vi "Supplementary Fig.15-2.vi"() -> ()   [LabVIEW 2018]
panel:
  out "files":string[](array[string])=["3rd-no3_th0_20191112171700-ext.FIRE", "3rd-no3_th0_20191112171706-ext.FIRE", "3rd-no3_th0_20191112171712-ext.FIRE", "3rd-no3_th0_20191112171717-ext.FIRE", "3rd-no3_th0_20191112171723-ext.FIRE", "3rd-no3_th0_20191112171728-ext.FIRE", "3rd-no3_th0_20191112171733-ext.FIRE", "3rd-no3_th0_20191112171739-ext.FIRE", "3rd-no3_th0_20191112171744-ext.FIRE", "3rd-no3_th0_20191112171750-ext.FIRE", "3rd-no3_th0_20191112171756-ext.FIRE", "3rd-no3_th0_20191112171801-ext.FIRE", "3rd-no3_th0_20191112171807-ext.FIRE", "3rd-no3_th0_20191112171813-ext.FIRE", "3rd-no3_th0_20191112171819-ext.FIRE", "3rd-no3_th0_20191112171824-ext.FIRE", "3rd-no3_th0_20191112171829-ext.FIRE", "3rd-no3_th0_20191112171835-ext.FIRE", "3rd-no3_th0_20191112171840-ext.FIRE", "3rd-no3_th0_20191112171846-ext.FIRE", "3rd-no3_th0_20191112171851-ext.FIRE", "3rd-no3_th0_20191112171857-ext.FIRE"]
  out "widths [um] (red x, red y, green x, green y)":dbl[][](array[numeric])
  in  "Array 3":T1(array[cluster])=[{"index"=6, "upper limit"=3.0, "lower limit"=1e-06, "Boolean"=TRUE}, {"index"=10, "upper limit"=3.0, "lower limit"=1e-06, "Boolean"=TRUE}, {"index"=14, "upper limit"=3.0, "lower limit"=1e-06, "Boolean"=TRUE}, {"index"=18, "upper limit"=3.0, "lower limit"=1e-06, "Boolean"=TRUE}]
  in  "file type":string=".info"
  in  "filepath (.info)":path
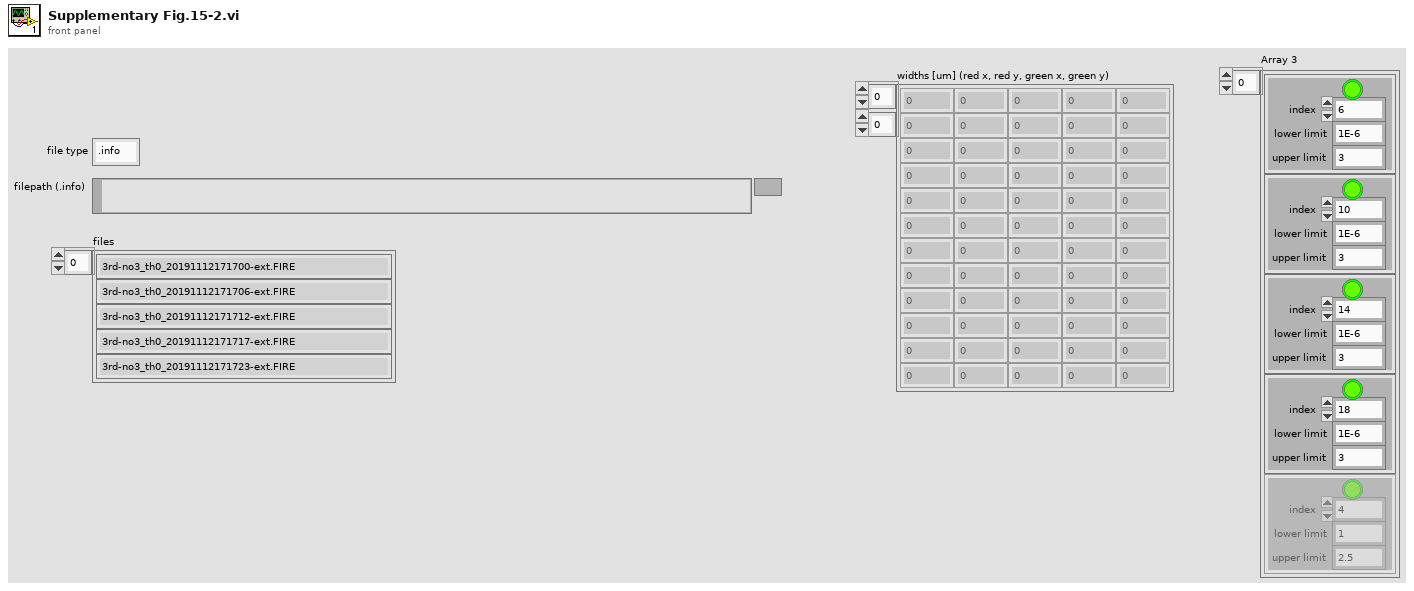
[diagram p1: front panel]
types:
  T1 = cluster{"index":i32, "upper limit":dbl, "lower limit":dbl, "Boolean":bool}[]
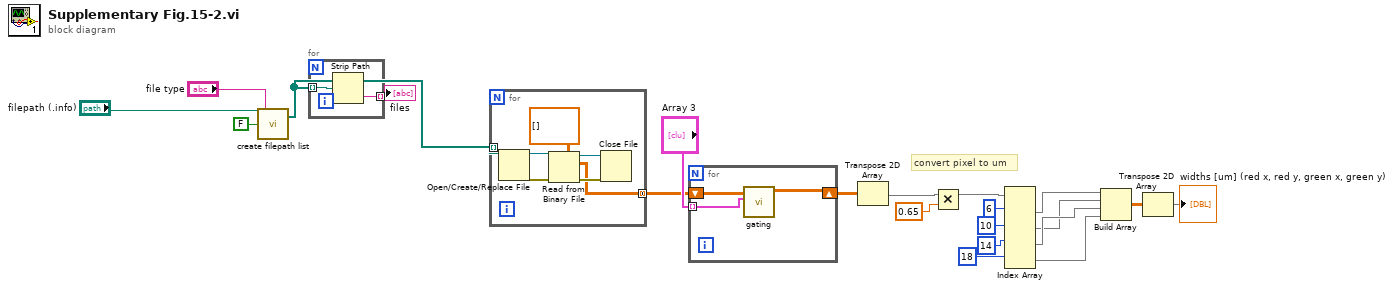
[diagram p0: block diagram]
diagram:
  # "convert pixel to um"
  n1 = call "create filepath list.vi"("regular expression"="file type", "search subholder"=FALSE, "path"="filepath (.info)") -> ("Array"=w19:path[])  [unwired: 1 out]
  n2 = for {
    tunnel: w19 -> [w23] mode=indexing
    tunnel: [w22] -> w1 mode=indexing
    n3 = Strip Path(path=w23) -> (name=w22:string)  [unwired: 1 out]
  }
  "files" <- w1
  n4 = for {
    tunnel: [w25] -> w4 mode=concatenating
    tunnel: w19 -> [w24] mode=indexing
    n5 = Open/Create/Replace File(file path (use dialog)=w24) -> (refnum out=w28:refnum<file>, error out=w27:errorcluster)  [unwired: 5 in, 1 out]
    n6 = Read from Binary File(5:dbl[][] [], 8:w27, 11:w28) -> (0:w30:errorcluster, 2:w25:dbl[][], 3:w29:refnum<file>)  [unwired: 3 in, 1 out]
    n7 = Close File(refnum=w29, error in=w30) -> ()  [unwired: 2 out]
  }
  n8 = for {
    shift-right: [w33] -> w21
    shift-left: w4 -> [w32]
    tunnel: "Array 3" -> [w31] mode=indexing
    n9 = call "gating.vi"("Cluster"=w31, "Array in"=w32) -> ("Array out"=w33:dbl[][])  [unwired: 8 in, 1 out]
  }
  n10 = Transpose 2D Array(2D array=w21) -> (transposed array=w9:dbl[][])
  n11 = Multiply(x=w9, y=0.65) -> (x*y=w17:dbl[][])
  n12 = Index Array(array=w17, index (row) #1=6 ("index (row)"), index (row) #2=10 ("index (row)"), index (row) #3=14 ("index (row)"), index (row) #4=18 ("index (row)")) -> (element #1=w11:dbl[], element #2=w12:dbl[], element #3=w13:dbl[], element #4=w14:dbl[])  [unwired: 4 in]
  n13 = Build Array(w11, w12, w13, w14) -> (w15:dbl[][])
  n14 = Transpose 2D Array(2D array=w15) -> (transposed array=→"widths [um] (red x, red y, green x, green y)":dbl[][])
